vi "getparam.vi"(8 "error in (no error)":errorcluster, 11 "Input":string="34,45,89") -> (0 "error out":errorcluster, 3 "Output":string)   [LabVIEW 2014]
uses:
  <userlib>/Nanonis Prog Interface V5/Scan/Piezos/Piezo Calibration Range Get.vi
  <userlib>/Nanonis Prog Interface V5/Nanonis Prog Interface.lvlib
panel:
  out "size(s)":i32=3
  # "."
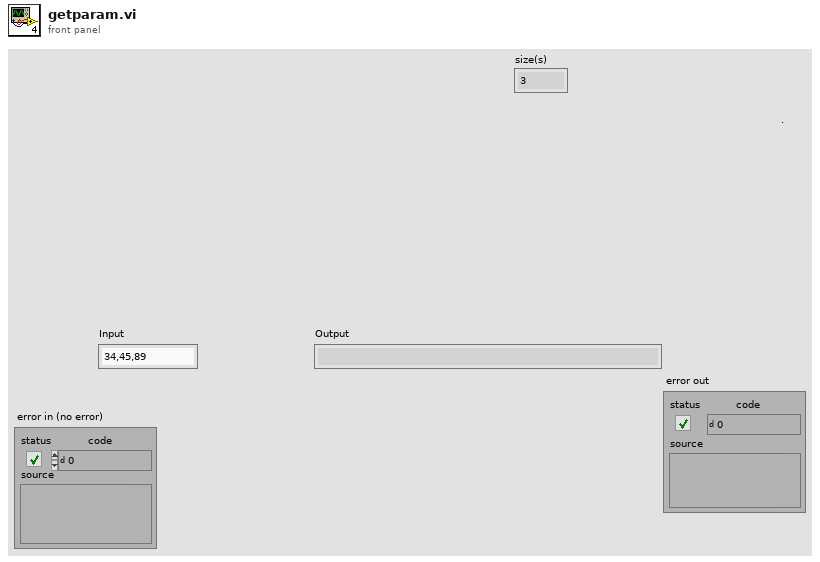
[diagram p1: front panel]
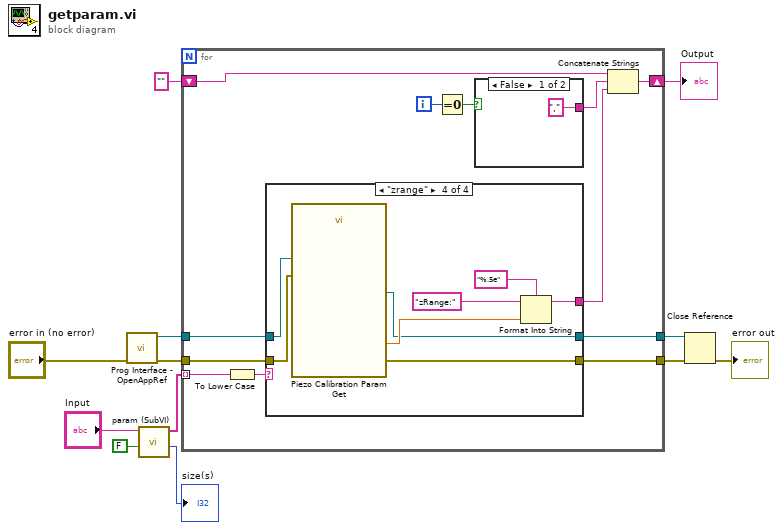
[diagram p0: block diagram]
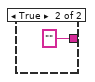
[diagram p2: hidden frame]
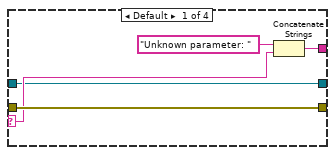
[diagram p3: hidden frame]
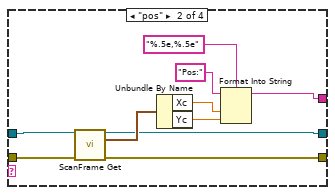
[diagram p4: hidden frame]
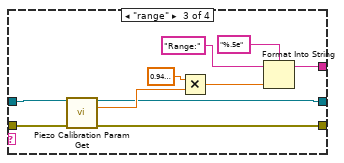
[diagram p5: hidden frame]
diagram:
  n1 = call <userlib>:"Prog Interface - OpenAppRef.vi"("Error in (no error)"="error in (no error)") -> ("Error out"=w5:errorcluster, "Application reference"=w7:refnum<vi>)  [unwired: 5 in]
  n2 = call <userlib>:"param (SubVI).vi"("Numeric"=FALSE, "Input"="Input") -> ("num"=→"size(s)":i32, "Array"=w8:string[])  [unwired: 7 in, 1 out]
  n3 = for {
    tunnel: w8 -> [w24] mode=indexing
    tunnel: w7 -> [w23]
    shift-right: [w19] -> w4
    shift-left: "" -> [w22]
    tunnel: w5 -> [w18]
    tunnel: [w17] -> w2
    tunnel: [w13] -> w3
    i -> [w14]
    n4 = To Lower Case(string=w24) -> (all lower case string=w16:string)
    n5 = case shown="\"zrange\"" w16 {
      selector: w16 -> [w29 _ _ _]
      tunnel: w23 -> [w27 w41 w51 w59]
      tunnel: [w31 w34 w47 w56] -> w20
      tunnel: w18 -> [w30 w40 w46 w55]
      tunnel: [w30 w33 w45 w54] -> w17
      tunnel: [w27 w32 w42 w52] -> w13
      frame Default {
        n6 = Concatenate Strings("Unknown parameter: " ("string"), w29) -> (w31:string)
      }
      frame "pos" {
        n7 = call <userlib>:"ScanFrame Get.vi"("Application ref in"=w41, "error in (no error)"=w40) -> ("Application ref out"=w32:refnum<vi>, "Center coordinates (m)"=w39:cluster{"Xc":sgl, "Yc":sgl}, "error out"=w33:errorcluster)  [unwired: 9 in, 2 out]
        n8 = Unbundle By Name(w39) -> ("Xc"=w36:sgl, "Yc"=w35:sgl)
        n9 = Format Into String(format string="%.5e,%.5e", initial string="Pos:", w36, w35) -> (resulting string=w34:string)  [unwired: 1 in, 1 out]
      }
      frame "range" {
        n10 = call-poly <userlib>:"Piezo Calibration Param Get.vi"("Application ref in"=w51, "error in (no error)"=w46) -> ("Application ref out"=w42:refnum<vi>, "Range X (m)"=w49:sgl, "error out"=w45:errorcluster)  [unwired: 9 in, 2 out]
        n11 = Multiply(x=sgl 0.95, y=w49) -> (x*y=w44:sgl)
        n12 = Format Into String(format string="%.5e", initial string="Range:", w44) -> (resulting string=w47:string)  [unwired: 1 in, 1 out]
      }
      frame "zrange" {
        n13 = call-poly <userlib>:"Piezo Calibration Param Get.vi"("Application ref in"=w59, "error in (no error)"=w55) -> ("Application ref out"=w52:refnum<vi>, "Range Z (m)"=w53:sgl, "error out"=w54:errorcluster)  [unwired: 9 in, 2 out]
        n14 = Format Into String(format string="%.5e", initial string="zRange:", w53) -> (resulting string=w56:string)  [unwired: 1 in, 1 out]
      }
    }
    n15 = Equal To 0?(x=w14) -> (x = 0?=w15:bool)
    n16 = case shown="False" w15 {
      tunnel: ["," ("string") "" ("string")] -> w21
      frame False {
      }
      frame True {
      }
    }
    n17 = Concatenate Strings(w22, w21, w20) -> (w19:string)
  }
  "Output" <- w4
  n18 = Close Reference(reference=w3, error in (no error)=w2) -> (error out=→"error out":errorcluster)
